vi "DeleteEventRefFile.vi"(8 "error in (no error)":errorcluster, 11 "data":variant) -> (0 "error out":errorcluster)   [LabVIEW 2017, in "FileManager.lvlib"]
uses:
  <vilib>/addons/InsightCM/Devices/Shared/Common/FileManager/FileManager.lvlib
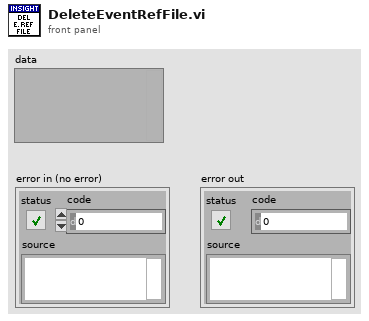
[diagram p1: front panel]
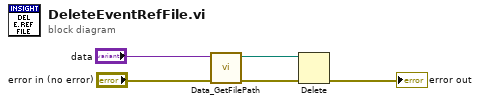
[diagram p0: block diagram]
diagram:
  n1 = call <vilib>:"Data_GetFilePath.vi"("error in (no error)"="error in (no error)", "data"="data") -> ("error out"=w3:errorcluster, "path"=w2:path)  [unwired: 8 in]
  n2 = Delete(path (use dialog)=w2, error in=w3) -> (error out=→"error out":errorcluster)  [unwired: 3 in, 2 out]
